vi "Shift Calculation_4.vi"(8 "error in (no error)":errorcluster, 9 "Current Time":timestamp, 10 "Time Stamp Out":timestamp[](array[timestamp])) -> (0 "error out":errorcluster, 2 "Shift":i32)   [LabVIEW 2017]
panel:
  in  "Shift Time Details":T1 {"3End" format="%<%H:%M:%S\n%x>T"; "2End" format="%<%H:%M:%S\n%x>T"; "3Start" format="%<%H:%M:%S\n%x>T"; "2Start" format="%<%H:%M:%S\n%x>T"; "1End" format="%<%H:%M:%S\n%x>T"; "1Start" format="%<%H:%M:%S\n%x>T"}
  # "Start Time"
  # "End Time"
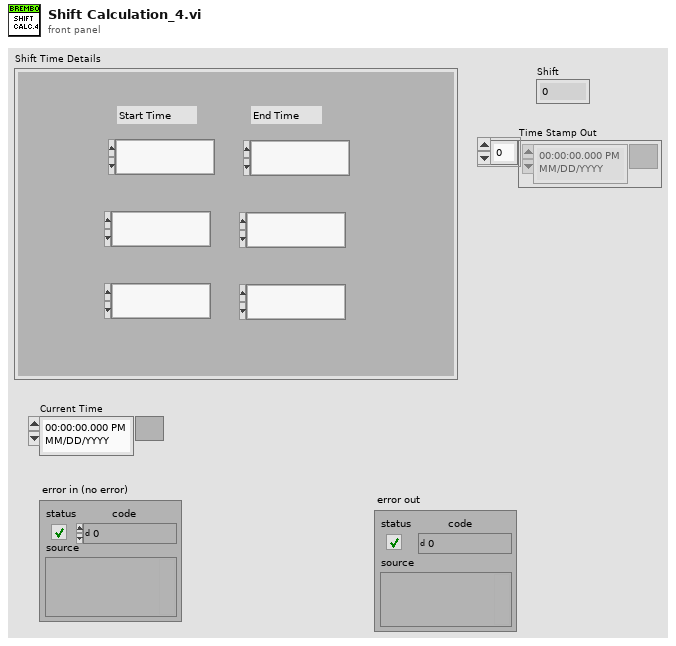
[diagram p1: front panel]
types:
  T1 = cluster{"1Start":timestamp, "1End":timestamp, "2Start":timestamp, "3Start":timestamp, "2End":timestamp, "3End":timestamp}
  T2 = typedef "LVDateTimeRec.ctl" = cluster{"fractional second":dbl, "second":i32, "minute":i32, "hour":i32, "day of month":i32, "month":i32, "year":i32, "day of week":i32, "day of year":i32, "DST":i32}
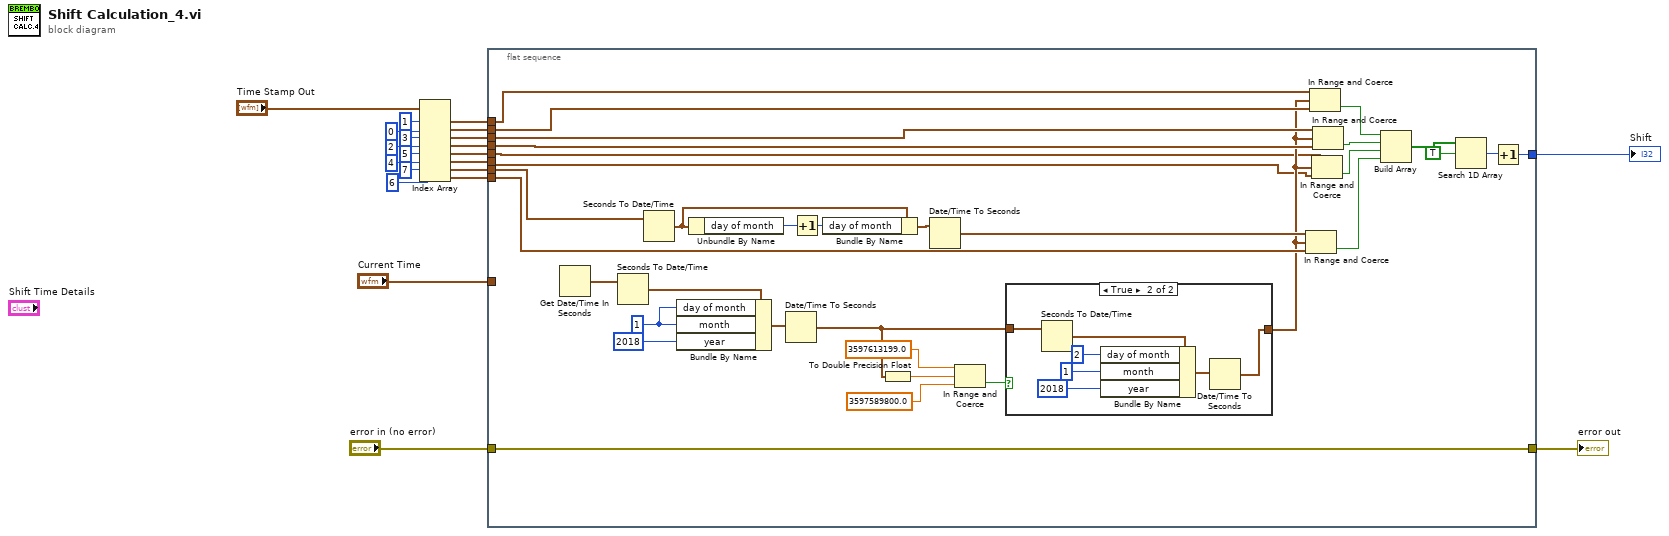
[diagram p0: block diagram]
diagram:
  n1 = Index Array(array="Time Stamp Out", index #1=1 ("index"), index #2=0 ("index"), index #3=3 ("index"), index #4=2 ("index"), index #5=5 ("index"), index #6=4 ("index"), index #7=7 ("index"), index #8=6 ("index")) -> (element #1=w14:timestamp, element #2=w13:timestamp, element #3=w10:timestamp, element #4=w9:timestamp, element #5=w6:timestamp, element #6=w5:timestamp, element #7=w2:timestamp, element #8=w1:timestamp)
  n2 = flat-sequence {
    tunnel: [w44] -> w21
    tunnel: "error in (no error)" -> [w34]
    tunnel: [w34] -> w19
    tunnel: "Current Time" -> [_]
    tunnel: w14 -> [w33]
    tunnel: w13 -> [w32]
    tunnel: w10 -> [w31]
    tunnel: w9 -> [w30]
    tunnel: w6 -> [w25]
    tunnel: w5 -> [w24]
    tunnel: w2 -> [w27]
    tunnel: w1 -> [w28]
    frame #0 {
      w37 = 1 ("day of month")
      n3 = Get Date/Time In Seconds() -> (seconds since 1Jan1904=w29:timestamp)
      n4 = Seconds To Date/Time(time stamp (now)=w29) -> (date time rec=w41:T2)  [unwired: 1 in]
      n5 = Seconds To Date/Time(time stamp (now)=w27) -> (date time rec=w53:T2)  [unwired: 1 in]
      n6 = Bundle By Name(cluster=w41, "day of month"=w37, "month"=w37, "year"=2018) -> (w43:T2)
      n7 = Unbundle By Name(w53) -> ("day of month"=w51:i32)
      n8 = Date/Time To Seconds(2:w43) -> (0:w35:timestamp)  [unwired: 1 in]
      n9 = Increment(x=w51) -> (x+1=w52:i32)
      n10 = Bundle By Name(cluster=w53, "day of month"=w52) -> (w54:T2)
      n11 = To Double Precision Float(number=w35) -> (double precision float=w38:dbl)
      n12 = Date/Time To Seconds(2:w54) -> (0:w50:timestamp)  [unwired: 1 in]
      n13 = In Range and Coerce(upper limit=3597613199.0 ("double precision float 2"), x=w38, lower limit=3597589800.0 ("double precision float")) -> (In Range?=w36:bool)  [unwired: 1 out]
      n14 = case shown="True" w36 {
        tunnel: w35 -> [w55 w58]
        tunnel: [w55 w57] -> w26
        frame False {
        }
        frame True {
          n15 = Seconds To Date/Time(time stamp (now)=w58) -> (date time rec=w60:T2)  [unwired: 1 in]
          n16 = Bundle By Name(cluster=w60, "day of month"=2, "month"=1 ("day of month"), "year"=2018) -> (w62:T2)
          n17 = Date/Time To Seconds(2:w62) -> (0:w57:timestamp)  [unwired: 1 in]
        }
      }
      n18 = In Range and Coerce(upper limit=w50, x=w26, lower limit=w28) -> (In Range?=w23:bool)  [unwired: 1 out]
      n19 = In Range and Coerce(upper limit=w33, x=w26, lower limit=w32) -> (In Range?=w49:bool)  [unwired: 1 out]
      n20 = In Range and Coerce(upper limit=w25, x=w26, lower limit=w24) -> (In Range?=w22:bool)  [unwired: 1 out]
      n21 = In Range and Coerce(upper limit=w31, x=w26, lower limit=w30) -> (In Range?=w48:bool)  [unwired: 1 out]
      n22 = Build Array(w49, w48, w22, w23) -> (w47:bool[])
      n23 = Search 1D Array(1D array=w47, element=TRUE) -> (index of element=w45:i32)  [unwired: 1 in]
      n24 = Increment(x=w45) -> (x+1=w44:i32)
    }
  }
  "Shift" <- w21
  "error out" <- w19
